vi "tls close.vi"(8 "error in":errorcluster, 11 "tls context":u64) -> (0 "error out":errorcluster, 3 "return":i32)   [LabVIEW 2016, in "lv tls dll.lvlib"]
uses:
  lv tls dll.lvlib
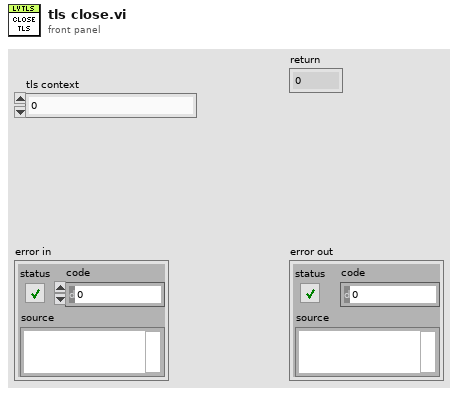
[diagram p1: front panel]
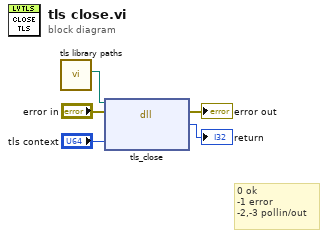
[diagram p0: block diagram]
diagram:
  # "0 ok\n-1 error\n-2,-3 pollin/out"
  n1 = call "tls library paths.vi"() -> ("libtls"=w4:path)  [unwired: 8 in, 3 out]
  n2 = dll-call lib="C:/Users/IEUser/Desktop/tlssimple/libtls-15.dll" fn="tls_close"(path in=w4, error in="error in", "context"="tls context") -> (error out=→"error out":errorcluster, "ret"=→"return":i32)  [unwired: 2 in, 1 out]
